vi "S4GUI_001.vi"() -> ()   [LabVIEW 2018] (continued)
                # "obsType"
                n1586 = call-dynamic "Read AcquisitionD.vi"("error in (no error)"=w3637, "S4ACS_GUI in"=w3638) -> ("error out"=w3627:errorcluster, "Acquisition.lvclass"=w3626:refnum<class "Acquisition.lvclass">, "S4ACS_GUI out"=w3616:refnum<class "S4GUI.lvclass">)  [unwired: 7 in]
                n1587 = local read "Exptime ch4"() -> (w3588:dbl)
                n1588 = call-dynamic "Read Channel.vi"("error in (no error)"=w3627, "Acquisition in"=w3626) -> ("error out"=w3624:errorcluster, "Channel.lvclass"=w3625:refnum<class "Channel.lvclass">, "Acquisition out"=w3615:refnum<class "Acquisition.lvclass">)  [unwired: 7 in]
                n1589 = call-dynamic "Read Interface.vi"("error in (no error)"=w3624, "Channel in"=w3625) -> ("error out"=w3633:errorcluster, "Interface.lvclass"=w3622:refnum<class "Interface.lvclass">, "Channel out"=w3623:refnum<class "Channel.lvclass">)  [unwired: 7 in]
                n1590 = call "Write Exposure Time.vi"("error in (no error)"=w3633, "Exposure Time"=w3588, "Interface in"=w3622) -> ("error out"=w3590:errorcluster, "Interface out"=w3592:refnum<class "Interface.lvclass">)  [unwired: 7 in]
                n1591 = case shown="Default" w3587 {
                  tunnel: w3592 -> [w3640 w3645]
                  tunnel: [w3640 w3644] -> w3591
                  tunnel: [w3639 w3643] -> w3589
                  tunnel: w3590 -> [w3639 w3642]
                  tunnel: w3588 -> [_ w3641]
                  frame "ZERO" {
                  }
                  frame Default {
                    n1592 = call-dynamic "Write prev ExpTime.vi"("error in (no error)"=w3642, "prev ExpTime"=w3641, "Interface in"=w3645) -> ("error out"=w3643:errorcluster, "Interface out"=w3644:refnum<class "Interface.lvclass">)  [unwired: 7 in]
                  }
                }
                n1593 = call-dynamic "Write Suffix.vi"("error in (no error)"=w3589, "Suffix"=w3634, "Interface in"=w3591) -> ("error out"=w3632:errorcluster, "Interface out"=w3621:refnum<class "Interface.lvclass">)  [unwired: 7 in]
                n1594 = call-dynamic "Write ObsType.vi"("error in (no error)"=w3632, "ObsType"=w3607, "Interface in"=w3621) -> ("error out"=w3631:errorcluster, "Interface out"=w3620:refnum<class "Interface.lvclass">)  [unwired: 7 in]
                n1595 = call-dynamic "Write Object.vi"("error in (no error)"=w3631, "Object"=w3606, "Interface in"=w3620) -> ("error out"=w3630:errorcluster, "Interface out"=w3619:refnum<class "Interface.lvclass">)  [unwired: 7 in]
                n1596 = call-dynamic "Write Comments.vi"("error in (no error)"=w3630, "Comments"=w3608, "Interface in"=w3619) -> ("error out"=w3629:errorcluster, "Interface out"=w3618:refnum<class "Interface.lvclass">)  [unwired: 7 in]
                n1597 = call-dynamic "Write DS9.vi"("error in (no error)"=w3629, "DS9"="F", "Interface in"=w3618) -> ("error out"=w3603:errorcluster, "Interface out"=w3605:refnum<class "Interface.lvclass">)  [unwired: 7 in]
                n1598 = property on="Exposure Time ch4" class="Slide (strict)"("Scale.Maximum"=w3588, "Scale.Minimum"=0.0 ("Scale.Range:Minimum")) -> ()  [unwired: 2 in, 2 out]
                n1599 = local read "Exp ch4"() -> (w3611:u32)
                n1600 = call-dynamic "Write Observer.vi"("error in (no error)"=w3603, "Observer"=w3601, "Interface in"=w3605) -> ("error out"=w3602:errorcluster, "Interface out"=w3604:refnum<class "Interface.lvclass">)  [unwired: 7 in]
                n1601 = property on="Exposure Done ch4" class="Slide (strict)"("Scale.Maximum"=w3611, "Scale.Minimum"=0.0 ("Scale.Range:Minimum")) -> ()  [unwired: 2 in, 2 out]
                n1602 = call-dynamic "Write # Images.vi"("error in (no error)"=w3602, "# Images"=w3611, "Interface in"=w3604) -> ("error out"=w3628:errorcluster, "Interface out"=w3617:refnum<class "Interface.lvclass">)  [unwired: 7 in]
                n1603 = call-dynamic "Write Interface.vi"("error in (no error)"=w3628, "Interface.lvclass"=w3617, "Channel in"=w3623) -> ("error out"=w3600:errorcluster, "Channel out"=w3599:refnum<class "Channel.lvclass">)  [unwired: 7 in]
                n1604 = call-dynamic "Write ciclos.vi"("error in (no error)"=w3600, "ciclos"=w3598, "Channel in"=w3599) -> ("error out"=w3596:errorcluster, "Channel out"=w3597:refnum<class "Channel.lvclass">)  [unwired: 7 in]
                n1605 = call-dynamic "Write sequencias.vi"("error in (no error)"=w3596, "sequencias"=w3593, "Channel in"=w3597) -> ("error out"=w3595:errorcluster, "Channel out"=w3594:refnum<class "Channel.lvclass">)  [unwired: 7 in]
                n1606 = call-dynamic "Write Channel.vi"("error in (no error)"=w3595, "Channel.lvclass"=w3594, "Acquisition in"=w3615) -> ("error out"=w3613:errorcluster, "Acquisition out"=w3614:refnum<class "Acquisition.lvclass">)  [unwired: 7 in]
                n1607 = call-dynamic "Write AcquisitionD.vi"("error in (no error)"=w3613, "Acquisition.lvclass"=w3614, "S4ACS_GUI in"=w3616) -> ("error out"=w3635:errorcluster, "S4ACS_GUI out"=w3636:refnum<class "S4GUI.lvclass">)  [unwired: 7 in]
              }
            }
            n1608 = call-dynamic "Write sequencias.vi"("error in (no error)"=w3387, "sequencias"=w3383, "S4GUI in"=w3385) -> ("error out"=w3386:errorcluster, "S4GUI out"=w3384:refnum<class "S4GUI.lvclass">)  [unwired: 7 in]
            n1609 = call-dynamic "Write ciclos.vi"("error in (no error)"=w3386, "ciclos"=w3388, "S4ACS_GUI in"=w3384) -> ("error out"=w3390:errorcluster, "S4ACS_GUI out"=w3392:refnum<class "S4GUI.lvclass">)  [unwired: 7 in]
            n1610 = property on="#Cycles Done" class="Slide (strict)"("Scale.Maximum"=w3388, "Scale.Minimum"=0.0 ("Scale.Range:Minor Increment")) -> ()  [unwired: 2 in, 2 out]
            n1611 = call-dynamic "Write TotalCiclos.vi"("error in (no error)"=w3390, "TotalCiclos"=w3388, "S4GUI in"=w3392) -> ("error out"=w3389:errorcluster, "S4GUI out"=w3391:refnum<class "S4GUI.lvclass">)  [unwired: 7 in]
          }
        }
        n1612 = property on="Pause SM" class="Bool"(error in=w3251, "DisabledEnum"=T7."Enabled" ("Disabled")) -> (error out=w3250:errorcluster)  [unwired: 1 in, 1 out]
      }
      event "# Cycles": Value Change {
        w3646 = 0.0 ("Scale.Range:Minor Increment")
        n1613 = event-data() -> ("NewVal"=w3647:u32)  [unwired: 1 in]
        n1614 = call-dynamic "Write ciclos.vi"("error in (no error)"=w3650, "ciclos"=w3647, "S4ACS_GUI in"=w3651) -> ("error out"=w3649:errorcluster, "S4ACS_GUI out"=w3648:refnum<class "S4GUI.lvclass">)  [unwired: 7 in]
        n1615 = property on="#Cycles Done" class="Slide (strict)"("Scale.Maximum"=w3647, "Scale.Minimum"=w3646) -> ()  [unwired: 2 in, 2 out]
        n1616 = property on="Cycles Done ch2" class="Slide (strict)"("Scale.Maximum"=w3647, "Scale.Minimum"=w3646) -> ()  [unwired: 2 in, 2 out]
        n1617 = property on="Cycles Done ch4" class="Slide (strict)"("Scale.Maximum"=w3647, "Scale.Minimum"=w3646) -> ()  [unwired: 2 in, 2 out]
        n1618 = property on="Cycles Done ch1" class="Slide (strict)"("Scale.Maximum"=w3647, "Scale.Minimum"=w3646) -> ()  [unwired: 2 in, 2 out]
        n1619 = property on="Cycles Done ch3" class="Slide (strict)"("Scale.Maximum"=w3647, "Scale.Minimum"=w3646) -> ()  [unwired: 2 in, 2 out]
      }
      event "AllConfig": Value Change {
        n1620 = event-data() -> ()  [unwired: 1 in, 6 out]
        n1621 = call "Read Instrument.lvclass.vi"("error in (no error)"=w3656, "S4ACS_GUI in"=w3657) -> ("error out"=w3736:errorcluster, "Instrument.lvclass"=w3703:refnum<class "Instrument.lvclass">, "S4ACS_GUI out"=w3734:refnum<class "S4GUI.lvclass">)  [unwired: 7 in]
        n1622 = call "Read ASEL.vi"("error in (no error)"=w3736, "Instrument in"=w3703) -> ("error out"=w3728:errorcluster, "Opt_Selector.lvclass"=w3727:refnum<class "Opt_Selector.lvclass">, "Instrument out"=w3735:refnum<class "Instrument.lvclass">)  [unwired: 7 in]
        n1623 = call-dynamic "Read State Machine.vi"("error in (no error)"=w3728, "Device in"=w3727) -> ("error out"=w3731:errorcluster, "State Machine.lvclass"=w3733:refnum<class "State Machine.lvclass">, "Device out"=w3725:refnum<class "Opt_Selector.lvclass">)  [unwired: 7 in]
        n1624 = call "Next State.vi"("error in (no error)"=w3731, "New_State"=1, "State Machine in"=w3733) -> ("error out"=w3730:errorcluster, "State Machine out"=w3729:refnum<class "State Machine.lvclass">)  [unwired: 7 in]
        n1625 = call-dynamic "Write State Machine.vi"("error in (no error)"=w3730, "State Machine.lvclass"=w3729, "Device in"=w3725) -> ("error out"=w3724:errorcluster, "Device out"=w3726:refnum<class "Opt_Selector.lvclass">)  [unwired: 7 in]
        n1626 = call "Write ASEL.vi"("error in (no error)"=w3724, "Opt_Selector.lvclass"=w3726, "Instrument in"=w3735) -> ("error out"=w3686:errorcluster, "Instrument out"=w3702:refnum<class "Instrument.lvclass">)  [unwired: 7 in]
        n1627 = call "Read CALW.vi"("error in (no error)"=w3686, "Instrument in"=w3702) -> ("error out"=w3719:errorcluster, "Opt_Selector.lvclass"=w3720:refnum<class "Opt_Selector.lvclass">, "Instrument out"=w3701:refnum<class "Instrument.lvclass">)  [unwired: 7 in]
        n1628 = call-dynamic "Read State Machine.vi"("error in (no error)"=w3719, "Device in"=w3720) -> ("error out"=w3716:errorcluster, "State Machine.lvclass"=w3714:refnum<class "State Machine.lvclass">, "Device out"=w3722:refnum<class "Opt_Selector.lvclass">)  [unwired: 7 in]
        n1629 = call "Next State.vi"("error in (no error)"=w3716, "New_State"=1, "State Machine in"=w3714) -> ("error out"=w3717:errorcluster, "State Machine out"=w3718:refnum<class "State Machine.lvclass">)  [unwired: 7 in]
        n1630 = call-dynamic "Write State Machine.vi"("error in (no error)"=w3717, "State Machine.lvclass"=w3718, "Device in"=w3722) -> ("error out"=w3723:errorcluster, "Device out"=w3721:refnum<class "Opt_Selector.lvclass">)  [unwired: 7 in]
        n1631 = call "Write CALW.vi"("error in (no error)"=w3723, "Opt_Selector.lvclass"=w3721, "Instrument in"=w3701) -> ("error out"=w3685:errorcluster, "Instrument out"=w3700:refnum<class "Instrument.lvclass">)  [unwired: 7 in]
        n1632 = call "Read WPSEL.vi"("error in (no error)"=w3685, "Instrument in"=w3700) -> ("error out"=w3708:errorcluster, "Opt_Selector.lvclass"=w3707:refnum<class "Opt_Selector.lvclass">, "Instrument out"=w3699:refnum<class "Instrument.lvclass">)  [unwired: 7 in]
        n1633 = call-dynamic "Read State Machine.vi"("error in (no error)"=w3708, "Device in"=w3707) -> ("error out"=w3711:errorcluster, "State Machine.lvclass"=w3713:refnum<class "State Machine.lvclass">, "Device out"=w3705:refnum<class "Opt_Selector.lvclass">)  [unwired: 7 in]
        n1634 = call "Next State.vi"("error in (no error)"=w3711, "New_State"=1, "State Machine in"=w3713) -> ("error out"=w3710:errorcluster, "State Machine out"=w3709:refnum<class "State Machine.lvclass">)  [unwired: 7 in]
        n1635 = call-dynamic "Write State Machine.vi"("error in (no error)"=w3710, "State Machine.lvclass"=w3709, "Device in"=w3705) -> ("error out"=w3704:errorcluster, "Device out"=w3706:refnum<class "Opt_Selector.lvclass">)  [unwired: 7 in]
        n1636 = call "Write WPSEL.vi"("error in (no error)"=w3704, "Opt_Selector.lvclass"=w3706, "Instrument in"=w3699) -> ("error out"=w3684:errorcluster, "Instrument out"=w3688:refnum<class "Instrument.lvclass">)  [unwired: 7 in]
        n1637 = call "Read WPROT.vi"("error in (no error)"=w3684, "Instrument in"=w3688) -> ("error out"=w3694:errorcluster, "Opt_Selector.lvclass"=w3695:refnum<class "Opt_Selector.lvclass">, "Instrument out"=w3687:refnum<class "Instrument.lvclass">)  [unwired: 7 in]
        n1638 = call-dynamic "Read State Machine.vi"("error in (no error)"=w3694, "Device in"=w3695) -> ("error out"=w3691:errorcluster, "State Machine.lvclass"=w3689:refnum<class "State Machine.lvclass">, "Device out"=w3697:refnum<class "Opt_Selector.lvclass">)  [unwired: 7 in]
        n1639 = call "Next State.vi"("error in (no error)"=w3691, "New_State"=1, "State Machine in"=w3689) -> ("error out"=w3692:errorcluster, "State Machine out"=w3693:refnum<class "State Machine.lvclass">)  [unwired: 7 in]
        n1640 = call-dynamic "Write State Machine.vi"("error in (no error)"=w3692, "State Machine.lvclass"=w3693, "Device in"=w3697) -> ("error out"=w3698:errorcluster, "Device out"=w3696:refnum<class "Opt_Selector.lvclass">)  [unwired: 7 in]
        n1641 = call "Write WPROT.vi"("error in (no error)"=w3698, "Opt_Selector.lvclass"=w3696, "Instrument in"=w3687) -> ("error out"=w3660:errorcluster, "Instrument out"=w3661:refnum<class "Instrument.lvclass">)  [unwired: 7 in]
        n1642 = call "Read GMIR.vi"("error in (no error)"=w3660, "Instrument in"=w3661) -> ("error out"=w3679:errorcluster, "Opt_Continuous.lvclass"=w3680:refnum<class "Opt_Continuous.lvclass">, "Instrument out"=w3673:refnum<class "Instrument.lvclass">)  [unwired: 7 in]
        n1643 = call-dynamic "Read State Machine.vi"("error in (no error)"=w3679, "Device in"=w3680) -> ("error out"=w3676:errorcluster, "State Machine.lvclass"=w3674:refnum<class "State Machine.lvclass">, "Device out"=w3682:refnum<class "Opt_Continuous.lvclass">)  [unwired: 7 in]
        n1644 = call "Next State.vi"("error in (no error)"=w3676, "New_State"=1, "State Machine in"=w3674) -> ("error out"=w3677:errorcluster, "State Machine out"=w3678:refnum<class "State Machine.lvclass">)  [unwired: 7 in]
        n1645 = call-dynamic "Write State Machine.vi"("error in (no error)"=w3677, "State Machine.lvclass"=w3678, "Device in"=w3682) -> ("error out"=w3683:errorcluster, "Device out"=w3681:refnum<class "Opt_Continuous.lvclass">)  [unwired: 7 in]
        n1646 = call "Write GMIR.vi"("error in (no error)"=w3683, "Opt_Continuous.lvclass"=w3681, "Instrument in"=w3673) -> ("error out"=w3658:errorcluster, "Instrument out"=w3659:refnum<class "Instrument.lvclass">)  [unwired: 7 in]
        n1647 = call "Read GFOC.vi"("error in (no error)"=w3658, "Instrument in"=w3659) -> ("error out"=w3668:errorcluster, "Opt_Continuous.lvclass"=w3669:refnum<class "Opt_Continuous.lvclass">, "Instrument out"=w3662:refnum<class "Instrument.lvclass">)  [unwired: 7 in]
        n1648 = call-dynamic "Read State Machine.vi"("error in (no error)"=w3668, "Device in"=w3669) -> ("error out"=w3665:errorcluster, "State Machine.lvclass"=w3663:refnum<class "State Machine.lvclass">, "Device out"=w3671:refnum<class "Opt_Continuous.lvclass">)  [unwired: 7 in]
        n1649 = call "Next State.vi"("error in (no error)"=w3665, "New_State"=1, "State Machine in"=w3663) -> ("error out"=w3666:errorcluster, "State Machine out"=w3667:refnum<class "State Machine.lvclass">)  [unwired: 7 in]
        n1650 = call-dynamic "Write State Machine.vi"("error in (no error)"=w3666, "State Machine.lvclass"=w3667, "Device in"=w3671) -> ("error out"=w3672:errorcluster, "Device out"=w3670:refnum<class "Opt_Continuous.lvclass">)  [unwired: 7 in]
        n1651 = call "Write GFOC.vi"("error in (no error)"=w3672, "Opt_Continuous.lvclass"=w3670, "Instrument in"=w3662) -> ("error out"=w3654:errorcluster, "Instrument out"=w3655:refnum<class "Instrument.lvclass">)  [unwired: 7 in]
        n1652 = call "Write Instrument.lvclass.vi"("error in (no error)"=w3654, "Instrument.lvclass"=w3655, "S4ACS_GUI in"=w3734) -> ("error out"=w3653:errorcluster, "S4ACS_GUI out"=w3652:refnum<class "S4GUI.lvclass">)  [unwired: 7 in]
      }
      event "Tab Acq Type": Value Change {
        # "Tab for choosing EXPOSURE MODE: Object, Dflat, Sflat, Dark, Zero, Focus"
        n1653 = event-data() -> ("NewVal"=w3743:T1)  [unwired: 1 in]
        n1654 = local read "Observer"() -> (w3739:string)
        n1655 = case shown="\"ZERO\"" w3743 {
          tunnel: ["OBJECT" "FLAT" "FLAT" "DARK" "ZERO" "FOCUS"] -> w3737
          tunnel: [w3779 w3783 w3787 w3791 w3795 w3799] -> w3742
          tunnel: [w3778 w3782 w3786 w3790 w3794 w3798] -> w3741
          tunnel: [w3777 w3781 w3785 w3789 w3793 w3797] -> w3740
          frame "OBJECT", Default {
            n1656 = local read "Object_obj"() -> (w3779:string)
            n1657 = local read "OBJECT Comments"() -> (w3777:string)
            n1658 = local read "object suffix"() -> (w3778:string)
          }
          frame "DFLAT" {
            n1659 = local read "DFLAT Comments"() -> (w3781:string)
            n1660 = local read "Object_dflat"() -> (w3783:string)
            n1661 = local read "dflat suffix"() -> (w3782:string)
          }
          frame "SFLAT" {
            n1662 = local read "SFLAT Comments"() -> (w3785:string)
            n1663 = local read "Object_sflat"() -> (w3787:string)
            n1664 = local read "sflat suffix"() -> (w3786:string)
          }
          frame "DARK" {
            n1665 = local read "Object_dark"() -> (w3791:string)
            n1666 = local read "dark suffix"() -> (w3790:string)
            n1667 = local read "DARK Comments"() -> (w3789:string)
          }
          frame "ZERO" {
            n1668 = local read "ZERO Comments"() -> (w3793:string)
            n1669 = local read "Object_zero"() -> (w3795:string)
            n1670 = local read "zero suffix"() -> (w3794:string)
          }
          frame "FOCUS" {
            n1671 = local read "FOCUS Comments"() -> (w3797:string)
            n1672 = local read "Object_focus"() -> (w3799:string)
            n1673 = local read "focus suffix"() -> (w3798:string)
          }
        }
        n1674 = call-dynamic "Write ExpMode.vi"("error in (no error)"=w3746, "ExpMode"=w3743, "S4GUI in"=w3747) -> ("error out"=w3744:errorcluster, "S4GUI out"=w3745:refnum<class "S4GUI.lvclass">)  [unwired: 7 in]
        n1675 = call-dynamic "Read AcquisitionC.vi"("error in (no error)"=w3744, "S4ACS_GUI in"=w3745) -> ("error out"=w3750:errorcluster, "Acquisition.lvclass"=w3751:refnum<class "Acquisition.lvclass">)  [unwired: 7 in, 1 out]
        n1676 = call-dynamic "Read AcquisitionA.vi"("error in (no error)"=w3744, "S4ACS_GUI in"=w3745) -> ("error out"=w3754:errorcluster, "Acquisition.lvclass"=w3755:refnum<class "Acquisition.lvclass">, "S4ACS_GUI out"=w3776:refnum<class "S4GUI.lvclass">)  [unwired: 7 in]
        n1677 = call "Read AcquisitionB.vi"("error in (no error)"=w3744, "S4ACS_GUI in"=w3745) -> ("error out"=w3752:errorcluster, "Acquisition.lvclass"=w3753:refnum<class "Acquisition.lvclass">)  [unwired: 7 in, 1 out]
        n1678 = call-dynamic "Read AcquisitionD.vi"("error in (no error)"=w3744, "S4ACS_GUI in"=w3745) -> ("error out"=w3748:errorcluster, "Acquisition.lvclass"=w3749:refnum<class "Acquisition.lvclass">)  [unwired: 7 in, 1 out]
        n1679 = To Lower Case(string=w3741) -> (all lower case string=w3738:string)
        n1680 = case shown="\"ZERO\"" w3743 {
          tunnel: [w3834 w4159 w4512] -> w3775
          tunnel: [w3833 w4158 w4511] -> w3774
          tunnel: [w3832 w4157 w4510] -> w3770
          tunnel: [w3831 w4156 w4509] -> w3769
          tunnel: [w3830 w4155 w4508] -> w3759
          tunnel: [w3829 w4154 w4507] -> w3758
          tunnel: [w3828 w4153 w4506] -> w3757
          tunnel: [w3827 w4152 w4505] -> w3756
          tunnel: w3755 -> [w3826 w4151 w4504]
          tunnel: w3754 -> [w3825 w4150 w4503]
          tunnel: w3753 -> [w3811 w4137 w4490]
          tunnel: w3752 -> [w3810 w4136 w4489]
          tunnel: w3751 -> [w3809 w4135 w4488]
          tunnel: w3750 -> [w3808 w4134 w4487]
          tunnel: w3749 -> [w3807 w4133 w4486]
          tunnel: w3748 -> [w3806 w4132 w4485]
          tunnel: w3742 -> [w3803 w4131 w4484]
          tunnel: w3740 -> [w3804 w4130 w4483]
          tunnel: w3739 -> [w3805 w4129 w4482]
          tunnel: w3738 -> [w3802 w4128 w4481]
          tunnel: w3737 -> [w3801 w4127 w4480]
          frame "ZERO" {
            w3824 = 1e-05 ("Exptime ch1")
            # "ZERO: EXPTIME=1E-5 (mandatory), shutter automatically closed, save current FRAME_TRANSFER (prev_FT) and reset FRAME_TRANSFER."
            n1681 = call "Read connection.vi"("error in (no error)"=w3808, "Server in"=w3809) -> ("error out"=w3816:errorcluster, "connection"=w3815:bool, "Server out"=w3817:refnum<class "Acquisition.lvclass">)  [unwired: 7 in]
            n1682 = call "Read connection.vi"("error in (no error)"=w3810, "Server in"=w3811) -> ("error out"=w3819:errorcluster, "connection"=w3818:bool, "Server out"=w3820:refnum<class "Acquisition.lvclass">)  [unwired: 7 in]
            n1683 = call "Read connection.vi"("error in (no error)"=w3825, "Server in"=w3826) -> ("error out"=w3822:errorcluster, "connection"=w3821:bool, "Server out"=w3823:refnum<class "Acquisition.lvclass">)  [unwired: 7 in]
            n1684 = call "Read connection.vi"("error in (no error)"=w3806, "Server in"=w3807) -> ("error out"=w3813:errorcluster, "connection"=w3812:bool, "Server out"=w3814:refnum<class "Acquisition.lvclass">)  [unwired: 7 in]
            n1685 = case shown="True" w3818 {
              tunnel: w3820 -> [w3982 w4022]
              tunnel: w3819 -> [w3981 w4021]
              tunnel: [w3982 w4020] -> w3832
              tunnel: [w3981 w4019] -> w3831
              tunnel: w3805 -> [_ w3998]
              tunnel: w3804 -> [_ w3997]
              tunnel: w3803 -> [_ w3996]
              tunnel: w3802 -> [_ w3989]
              tunnel: w3801 -> [_ w3988]
              frame False {
              }
              frame True {
                # "nome do arquivo .cfg"
                # "seção no arquivo .cfg"
                n1686 = call-dynamic "Read Channel.vi"("error in (no error)"=w4021, "Acquisition in"=w4022) -> ("error out"=w4026:errorcluster, "Channel.lvclass"=w4025:refnum<class "Channel.lvclass">, "Acquisition out"=w4024:refnum<class "Acquisition.lvclass">)  [unwired: 7 in]
                n1687 = call-dynamic "Read Interface.vi"("error in (no error)"=w4026, "Channel in"=w4025) -> ("error out"=w3985:errorcluster, "Interface.lvclass"=w3986:refnum<class "Interface.lvclass">, "Channel out"=w4023:refnum<class "Channel.lvclass">)  [unwired: 7 in]
                n1688 = call-dynamic "Write restoreExpTime.vi"("error in (no error)"=w3985, "restoreExpTime"=TRUE, "Interface in"=w3986) -> ("error out"=w3983:errorcluster, "Interface out"=w3984:refnum<class "Interface.lvclass">)  [unwired: 7 in]
                n1689 = call-dynamic "Get CCD_Config.vi"("error in (no error)"=w3983, "Interface in"=w3984) -> ("error out"=w3992:errorcluster, "output cluster"=w3995:T24, "Interface out"=w3993:refnum<class "Interface.lvclass">)  [unwired: 7 in]
                n1690 = stacked-sequence {
                  tunnel: [_ w4052] -> w4030
                  tunnel: w3995 -> [_ w4051]
                  tunnel: w3995 -> [w4049 _]
                  tunnel: [w4048 _] -> w3990
                  frame #0 {
                    n1691 = Unbundle By Name(w4049) -> ("FRAME_TRANSFER"=w4048:bool)
                  }
                  frame #1 {
                    # "closed"
                    n1692 = Bundle By Name(cluster=w4051, "SHUTTER_MODE"=u8 2, "FRAME_TRANSFER"=FALSE) -> (w4052:T24)
                  }
                }
                n1693 = call-dynamic "Write PREV_FT.vi"("error in (no error)"=w3992, "PREV_FT"=w3990, "Interface in"=w3993) -> ("error out"=w3991:errorcluster, "Interface out"=w3994:refnum<class "Interface.lvclass">)  [unwired: 7 in]
                n1694 = call-dynamic "Set CCD_Config.vi"("error in (no error)"=w3991, "input cluster"=w4030, "Interface in"=w3994) -> ("error out"=w4029:errorcluster, "Interface out"=w4031:refnum<class "Interface.lvclass">)  [unwired: 7 in]
                n1695 = Flatten To String(anything=w4030, error in (no error)=w4029) -> (data string=w4027:string, error out=w4028:errorcluster)  [unwired: 2 in, 1 out]
                n1696 = call "Write flatted cluster.vi"("error in (no error)"=w4028, "flatted cluster"=w4027, "Interface in"=w4031) -> ("error out"=w4033:errorcluster, "Interface out"=w4032:refnum<class "Interface.lvclass">)  [unwired: 7 in]
                n1697 = call-dynamic "Write Interface.vi"("error in (no error)"=w4033, "Interface.lvclass"=w4032, "Channel in"=w4023) -> ("error out"=w4038:errorcluster, "Channel out"=w4039:refnum<class "Channel.lvclass">)  [unwired: 7 in]
                n1698 = call "Write section_name.vi"("error in (no error)"=w4038, "section_name"="CCD_ACS2", "Channel in"=w4039) -> ("error out"=w4037:errorcluster, "Channel out"=w4042:refnum<class "Channel.lvclass">)  [unwired: 7 in]
                n1699 = call-dynamic "save config.vi"("error in (no error)"=w4037, "file config"="lastsaved.cfg", "Channel in"=w4042) -> ("error out"=w4001:errorcluster, "Channel out"=w4002:refnum<class "Channel.lvclass">)  [unwired: 7 in]
                n1700 = local read "Filter2"() -> (w4003:u8)
                n1701 = call-dynamic "Write Filter.vi"("error in (no error)"=w4001, "Filter"=w4003, "Channel in"=w4002) -> ("error out"=w4010:errorcluster, "Channel out"=w4011:refnum<class "Channel.lvclass">)  [unwired: 7 in]
                n1702 = call-dynamic "Read Interface.vi"("error in (no error)"=w4010, "Channel in"=w4011) -> ("error out"=w4008:errorcluster, "Interface.lvclass"=w4013:refnum<class "Interface.lvclass">, "Channel out"=w4012:refnum<class "Channel.lvclass">)  [unwired: 7 in]
                n1703 = call-dynamic "Write Suffix.vi"("error in (no error)"=w4008, "Suffix"=w3989, "Interface in"=w4013) -> ("error out"=w4004:errorcluster, "Interface out"=w4014:refnum<class "Interface.lvclass">)  [unwired: 7 in]
                n1704 = call-dynamic "Write ObsType.vi"("error in (no error)"=w4004, "ObsType"=w3988, "Interface in"=w4014) -> ("error out"=w4005:errorcluster, "Interface out"=w4015:refnum<class "Interface.lvclass">)  [unwired: 7 in]
                n1705 = call-dynamic "Write Object.vi"("error in (no error)"=w4005, "Object"=w3996, "Interface in"=w4015) -> ("error out"=w4006:errorcluster, "Interface out"=w4016:refnum<class "Interface.lvclass">)  [unwired: 7 in]
                n1706 = call-dynamic "Write Comments.vi"("error in (no error)"=w4006, "Comments"=w3997, "Interface in"=w4016) -> ("error out"=w4007:errorcluster, "Interface out"=w4017:refnum<class "Interface.lvclass">)  [unwired: 7 in]
                n1707 = call-dynamic "Write Observer.vi"("error in (no error)"=w4007, "Observer"=w3998, "Interface in"=w4017) -> ("error out"=w4009:errorcluster, "Interface out"=w4018:refnum<class "Interface.lvclass">)  [unwired: 7 in]
                n1708 = call-dynamic "Write Interface.vi"("error in (no error)"=w4009, "Interface.lvclass"=w4018, "Channel in"=w4012) -> ("error out"=w4000:errorcluster, "Channel out"=w3999:refnum<class "Channel.lvclass">)  [unwired: 7 in]
                n1709 = call-dynamic "Read State Machine.vi"("error in (no error)"=w4000, "Device in"=w3999) -> ("error out"=w4034:errorcluster, "State Machine.lvclass"=w4044:refnum<class "State Machine.lvclass">, "Device out"=w4043:refnum<class "Channel.lvclass">)  [unwired: 7 in]
                n1710 = call-dynamic "Write State.vi"("error in (no error)"=w4034, "State"=60, "State Machine in"=w4044) -> ("error out"=w4035:errorcluster, "State Machine out"=w4045:refnum<class "State Machine.lvclass">)  [unwired: 7 in]
                n1711 = call-dynamic "Write State Machine.vi"("error in (no error)"=w4035, "State Machine.lvclass"=w4045, "Device in"=w4043) -> ("error out"=w4047:errorcluster, "Device out"=w4046:refnum<class "Channel.lvclass">)  [unwired: 7 in]
                n1712 = call-dynamic "Write Channel.vi"("error in (no error)"=w4047, "Channel.lvclass"=w4046, "Acquisition in"=w4024) -> ("error out"=w4019:errorcluster, "Acquisition out"=w4020:refnum<class "Acquisition.lvclass">)  [unwired: 7 in]
              }
            }
            n1713 = case shown="True" w3821 {
              tunnel: [w4054 w4116] -> w3833
              tunnel: [w4055 w4115] -> w3834
              tunnel: w3823 -> [w4055 w4093]
              tunnel: w3822 -> [w4054 w4092]
              tunnel: w3805 -> [_ w4071]
              tunnel: w3804 -> [_ w4070]
              tunnel: w3803 -> [_ w4069]
              tunnel: w3802 -> [_ w4062]
              tunnel: w3801 -> [_ w4061]
              frame False {
              }
              frame True {
                # "nome do arquivo .cfg"
                # "seção no arquivo .cfg"
                n1714 = call-dynamic "Read Channel.vi"("error in (no error)"=w4092, "Acquisition in"=w4093) -> ("error out"=w4117:errorcluster, "Channel.lvclass"=w4118:refnum<class "Channel.lvclass">, "Acquisition out"=w4119:refnum<class "Acquisition.lvclass">)  [unwired: 7 in]
                n1715 = call-dynamic "Read Interface.vi"("error in (no error)"=w4117, "Channel in"=w4118) -> ("error out"=w4058:errorcluster, "Interface.lvclass"=w4060:refnum<class "Interface.lvclass">, "Channel out"=w4120:refnum<class "Channel.lvclass">)  [unwired: 7 in]
                n1716 = call-dynamic "Write restoreExpTime.vi"("error in (no error)"=w4058, "restoreExpTime"=TRUE, "Interface in"=w4060) -> ("error out"=w4057:errorcluster, "Interface out"=w4059:refnum<class "Interface.lvclass">)  [unwired: 7 in]
                n1717 = call-dynamic "Get CCD_Config.vi"("error in (no error)"=w4057, "Interface in"=w4059) -> ("error out"=w4066:errorcluster, "output cluster"=w4064:T24, "Interface out"=w4068:refnum<class "Interface.lvclass">)  [unwired: 7 in]
                n1718 = stacked-sequence {
                  tunnel: [_ w4126] -> w4111
                  tunnel: w4064 -> [_ w4123]
                  tunnel: w4064 -> [w4122 _]
                  tunnel: [w4121 _] -> w4063
                  frame #0 {
                    n1719 = Unbundle By Name(w4122) -> ("FRAME_TRANSFER"=w4121:bool)
                  }
                  frame #1 {
                    # "closed"
                    n1720 = Bundle By Name(cluster=w4123, "SHUTTER_MODE"=u8 2, "FRAME_TRANSFER"=FALSE) -> (w4126:T24)
                  }
                }
                n1721 = call-dynamic "Write PREV_FT.vi"("error in (no error)"=w4066, "PREV_FT"=w4063, "Interface in"=w4068) -> ("error out"=w4065:errorcluster, "Interface out"=w4067:refnum<class "Interface.lvclass">)  [unwired: 7 in]
                n1722 = call-dynamic "Set CCD_Config.vi"("error in (no error)"=w4065, "input cluster"=w4111, "Interface in"=w4067) -> ("error out"=w4112:errorcluster, "Interface out"=w4110:refnum<class "Interface.lvclass">)  [unwired: 7 in]
                n1723 = Flatten To String(anything=w4111, error in (no error)=w4112) -> (data string=w4114:string, error out=w4113:errorcluster)  [unwired: 2 in, 1 out]
                n1724 = call "Write flatted cluster.vi"("error in (no error)"=w4113, "flatted cluster"=w4114, "Interface in"=w4110) -> ("error out"=w4108:errorcluster, "Interface out"=w4109:refnum<class "Interface.lvclass">)  [unwired: 7 in]
                n1725 = call-dynamic "Write Interface.vi"("error in (no error)"=w4108, "Interface.lvclass"=w4109, "Channel in"=w4120) -> ("error out"=w4103:errorcluster, "Channel out"=w4102:refnum<class "Channel.lvclass">)  [unwired: 7 in]
                n1726 = call "Write section_name.vi"("error in (no error)"=w4103, "section_name"="CCD_ACS1", "Channel in"=w4102) -> ("error out"=w4104:errorcluster, "Channel out"=w4099:refnum<class "Channel.lvclass">)  [unwired: 7 in]
                n1727 = call-dynamic "save config.vi"("error in (no error)"=w4104, "file config"="lastsaved.cfg", "Channel in"=w4099) -> ("error out"=w4082:errorcluster, "Channel out"=w4083:refnum<class "Channel.lvclass">)  [unwired: 7 in]
                n1728 = local read "Filter1"() -> (w4084:u8)
                n1729 = call-dynamic "Write Filter.vi"("error in (no error)"=w4082, "Filter"=w4084, "Channel in"=w4083) -> ("error out"=w4091:errorcluster, "Channel out"=w4081:refnum<class "Channel.lvclass">)  [unwired: 7 in]
                n1730 = call-dynamic "Read Interface.vi"("error in (no error)"=w4091, "Channel in"=w4081) -> ("error out"=w4089:errorcluster, "Interface.lvclass"=w4080:refnum<class "Interface.lvclass">, "Channel out"=w4074:refnum<class "Channel.lvclass">)  [unwired: 7 in]
                n1731 = call-dynamic "Write Suffix.vi"("error in (no error)"=w4089, "Suffix"=w4062, "Interface in"=w4080) -> ("error out"=w4085:errorcluster, "Interface out"=w4079:refnum<class "Interface.lvclass">)  [unwired: 7 in]
                n1732 = call-dynamic "Write ObsType.vi"("error in (no error)"=w4085, "ObsType"=w4061, "Interface in"=w4079) -> ("error out"=w4086:errorcluster, "Interface out"=w4078:refnum<class "Interface.lvclass">)  [unwired: 7 in]
                n1733 = call-dynamic "Write Object.vi"("error in (no error)"=w4086, "Object"=w4069, "Interface in"=w4078) -> ("error out"=w4087:errorcluster, "Interface out"=w4077:refnum<class "Interface.lvclass">)  [unwired: 7 in]
                n1734 = call-dynamic "Write Comments.vi"("error in (no error)"=w4087, "Comments"=w4070, "Interface in"=w4077) -> ("error out"=w4088:errorcluster, "Interface out"=w4076:refnum<class "Interface.lvclass">)  [unwired: 7 in]
                n1735 = call-dynamic "Write Observer.vi"("error in (no error)"=w4088, "Observer"=w4071, "Interface in"=w4076) -> ("error out"=w4090:errorcluster, "Interface out"=w4075:refnum<class "Interface.lvclass">)  [unwired: 7 in]
                n1736 = call-dynamic "Write Interface.vi"("error in (no error)"=w4090, "Interface.lvclass"=w4075, "Channel in"=w4074) -> ("error out"=w4072:errorcluster, "Channel out"=w4073:refnum<class "Channel.lvclass">)  [unwired: 7 in]
                n1737 = call-dynamic "Read State Machine.vi"("error in (no error)"=w4072, "Device in"=w4073) -> ("error out"=w4107:errorcluster, "State Machine.lvclass"=w4097:refnum<class "State Machine.lvclass">, "Device out"=w4098:refnum<class "Channel.lvclass">)  [unwired: 7 in]
                n1738 = call-dynamic "Write State.vi"("error in (no error)"=w4107, "State"=60, "State Machine in"=w4097) -> ("error out"=w4106:errorcluster, "State Machine out"=w4096:refnum<class "State Machine.lvclass">)  [unwired: 7 in]
                n1739 = call-dynamic "Write State Machine.vi"("error in (no error)"=w4106, "State Machine.lvclass"=w4096, "Device in"=w4098) -> ("error out"=w4094:errorcluster, "Device out"=w4095:refnum<class "Channel.lvclass">)  [unwired: 7 in]
                n1740 = call-dynamic "Write Channel.vi"("error in (no error)"=w4094, "Channel.lvclass"=w4095, "Acquisition in"=w4119) -> ("error out"=w4116:errorcluster, "Acquisition out"=w4115:refnum<class "Acquisition.lvclass">)  [unwired: 7 in]
              }
            }
            n1741 = case shown="True" w3815 {
              tunnel: w3817 -> [w3909 w3949]
              tunnel: w3816 -> [w3908 w3948]
              tunnel: [w3909 w3947] -> w3830
              tunnel: [w3908 w3946] -> w3829
              tunnel: w3805 -> [_ w3925]
              tunnel: w3804 -> [_ w3924]
              tunnel: w3803 -> [_ w3923]
              tunnel: w3802 -> [_ w3916]
              tunnel: w3801 -> [_ w3915]
              frame False {
              }
              frame True {
                # "nome do arquivo .cfg"
                # "seção no arquivo .cfg"
                n1742 = call-dynamic "Read Channel.vi"("error in (no error)"=w3948, "Acquisition in"=w3949) -> ("error out"=w3953:errorcluster, "Channel.lvclass"=w3952:refnum<class "Channel.lvclass">, "Acquisition out"=w3951:refnum<class "Acquisition.lvclass">)  [unwired: 7 in]
                n1743 = call-dynamic "Read Interface.vi"("error in (no error)"=w3953, "Channel in"=w3952) -> ("error out"=w3911:errorcluster, "Interface.lvclass"=w3913:refnum<class "Interface.lvclass">, "Channel out"=w3950:refnum<class "Channel.lvclass">)  [unwired: 7 in]
                n1744 = call-dynamic "Write restoreExpTime.vi"("error in (no error)"=w3911, "restoreExpTime"=TRUE, "Interface in"=w3913) -> ("error out"=w3910:errorcluster, "Interface out"=w3912:refnum<class "Interface.lvclass">)  [unwired: 7 in]
                n1745 = call-dynamic "Get CCD_Config.vi"("error in (no error)"=w3910, "Interface in"=w3912) -> ("error out"=w3918:errorcluster, "output cluster"=w3922:T24, "Interface out"=w3921:refnum<class "Interface.lvclass">)  [unwired: 7 in]
                n1746 = stacked-sequence {
                  tunnel: [_ w3979] -> w3957
                  tunnel: w3922 -> [_ w3978]
                  tunnel: w3922 -> [w3976 _]
                  tunnel: [w3975 _] -> w3917
                  frame #0 {
                    n1747 = Unbundle By Name(w3976) -> ("FRAME_TRANSFER"=w3975:bool)
                  }
                  frame #1 {
                    # "closed"
                    n1748 = Bundle By Name(cluster=w3978, "SHUTTER_MODE"=u8 2, "FRAME_TRANSFER"=FALSE) -> (w3979:T24)
                  }
                }
                n1749 = call-dynamic "Write PREV_FT.vi"("error in (no error)"=w3918, "PREV_FT"=w3917, "Interface in"=w3921) -> ("error out"=w3919:errorcluster, "Interface out"=w3920:refnum<class "Interface.lvclass">)  [unwired: 7 in]
                n1750 = call-dynamic "Set CCD_Config.vi"("error in (no error)"=w3919, "input cluster"=w3957, "Interface in"=w3920) -> ("error out"=w3956:errorcluster, "Interface out"=w3958:refnum<class "Interface.lvclass">)  [unwired: 7 in]
                n1751 = Flatten To String(anything=w3957, error in (no error)=w3956) -> (data string=w3954:string, error out=w3955:errorcluster)  [unwired: 2 in, 1 out]
                n1752 = call "Write flatted cluster.vi"("error in (no error)"=w3955, "flatted cluster"=w3954, "Interface in"=w3958) -> ("error out"=w3960:errorcluster, "Interface out"=w3959:refnum<class "Interface.lvclass">)  [unwired: 7 in]
                n1753 = call-dynamic "Write Interface.vi"("error in (no error)"=w3960, "Interface.lvclass"=w3959, "Channel in"=w3950) -> ("error out"=w3965:errorcluster, "Channel out"=w3966:refnum<class "Channel.lvclass">)  [unwired: 7 in]
                n1754 = call "Write section_name.vi"("error in (no error)"=w3965, "section_name"="CCD_ACS3", "Channel in"=w3966) -> ("error out"=w3964:errorcluster, "Channel out"=w3969:refnum<class "Channel.lvclass">)  [unwired: 7 in]
                n1755 = call-dynamic "save config.vi"("error in (no error)"=w3964, "file config"="lastsaved.cfg", "Channel in"=w3969) -> ("error out"=w3927:errorcluster, "Channel out"=w3929:refnum<class "Channel.lvclass">)  [unwired: 7 in]
                n1756 = local read "Filter3"() -> (w3945:u8)
                n1757 = call-dynamic "Write Filter.vi"("error in (no error)"=w3927, "Filter"=w3945, "Channel in"=w3929) -> ("error out"=w3938:errorcluster, "Channel out"=w3937:refnum<class "Channel.lvclass">)  [unwired: 7 in]
                n1758 = call-dynamic "Read Interface.vi"("error in (no error)"=w3938, "Channel in"=w3937) -> ("error out"=w3940:errorcluster, "Interface.lvclass"=w3935:refnum<class "Interface.lvclass">, "Channel out"=w3936:refnum<class "Channel.lvclass">)  [unwired: 7 in]
                n1759 = call-dynamic "Write Suffix.vi"("error in (no error)"=w3940, "Suffix"=w3916, "Interface in"=w3935) -> ("error out"=w3944:errorcluster, "Interface out"=w3934:refnum<class "Interface.lvclass">)  [unwired: 7 in]
                n1760 = call-dynamic "Write ObsType.vi"("error in (no error)"=w3944, "ObsType"=w3915, "Interface in"=w3934) -> ("error out"=w3943:errorcluster, "Interface out"=w3933:refnum<class "Interface.lvclass">)  [unwired: 7 in]
                n1761 = call-dynamic "Write Object.vi"("error in (no error)"=w3943, "Object"=w3923, "Interface in"=w3933) -> ("error out"=w3942:errorcluster, "Interface out"=w3932:refnum<class "Interface.lvclass">)  [unwired: 7 in]
                n1762 = call-dynamic "Write Comments.vi"("error in (no error)"=w3942, "Comments"=w3924, "Interface in"=w3932) -> ("error out"=w3941:errorcluster, "Interface out"=w3931:refnum<class "Interface.lvclass">)  [unwired: 7 in]
                n1763 = call-dynamic "Write Observer.vi"("error in (no error)"=w3941, "Observer"=w3925, "Interface in"=w3931) -> ("error out"=w3939:errorcluster, "Interface out"=w3930:refnum<class "Interface.lvclass">)  [unwired: 7 in]
                n1764 = call-dynamic "Write Interface.vi"("error in (no error)"=w3939, "Interface.lvclass"=w3930, "Channel in"=w3936) -> ("error out"=w3926:errorcluster, "Channel out"=w3928:refnum<class "Channel.lvclass">)  [unwired: 7 in]
                n1765 = call-dynamic "Read State Machine.vi"("error in (no error)"=w3926, "Device in"=w3928) -> ("error out"=w3961:errorcluster, "State Machine.lvclass"=w3971:refnum<class "State Machine.lvclass">, "Device out"=w3970:refnum<class "Channel.lvclass">)  [unwired: 7 in]
                n1766 = call-dynamic "Write State.vi"("error in (no error)"=w3961, "State"=60, "State Machine in"=w3971) -> ("error out"=w3962:errorcluster, "State Machine out"=w3972:refnum<class "State Machine.lvclass">)  [unwired: 7 in]
                n1767 = call-dynamic "Write State Machine.vi"("error in (no error)"=w3962, "State Machine.lvclass"=w3972, "Device in"=w3970) -> ("error out"=w3974:errorcluster, "Device out"=w3973:refnum<class "Channel.lvclass">)  [unwired: 7 in]
                n1768 = call-dynamic "Write Channel.vi"("error in (no error)"=w3974, "Channel.lvclass"=w3973, "Acquisition in"=w3951) -> ("error out"=w3946:errorcluster, "Acquisition out"=w3947:refnum<class "Acquisition.lvclass">)  [unwired: 7 in]
              }
            }
            n1769 = case shown="True" w3812 {
              tunnel: w3814 -> [w3836 w3876]
              tunnel: w3813 -> [w3835 w3875]
              tunnel: [w3836 w3874] -> w3828
              tunnel: [w3835 w3873] -> w3827
              tunnel: w3805 -> [_ w3852]
              tunnel: w3804 -> [_ w3851]
              tunnel: w3803 -> [_ w3850]
              tunnel: w3802 -> [_ w3843]
              tunnel: w3801 -> [_ w3842]
              frame False {
              }
              frame True {
                # "nome do arquivo .cfg"
                # "seção no arquivo .cfg"
                n1770 = call-dynamic "Read Channel.vi"("error in (no error)"=w3875, "Acquisition in"=w3876) -> ("error out"=w3898:errorcluster, "Channel.lvclass"=w3899:refnum<class "Channel.lvclass">, "Acquisition out"=w3900:refnum<class "Acquisition.lvclass">)  [unwired: 7 in]
                n1771 = call-dynamic "Read Interface.vi"("error in (no error)"=w3898, "Channel in"=w3899) -> ("error out"=w3840:errorcluster, "Interface.lvclass"=w3838:refnum<class "Interface.lvclass">, "Channel out"=w3901:refnum<class "Channel.lvclass">)  [unwired: 7 in]
                n1772 = call-dynamic "Write restoreExpTime.vi"("error in (no error)"=w3840, "restoreExpTime"=TRUE, "Interface in"=w3838) -> ("error out"=w3839:errorcluster, "Interface out"=w3837:refnum<class "Interface.lvclass">)  [unwired: 7 in]
                n1773 = call-dynamic "Get CCD_Config.vi"("error in (no error)"=w3839, "Interface in"=w3837) -> ("error out"=w3846:errorcluster, "output cluster"=w3849:T24, "Interface out"=w3845:refnum<class "Interface.lvclass">)  [unwired: 7 in]
                n1774 = stacked-sequence {
                  tunnel: w3849 -> [_ w3907]
                  tunnel: [_ w3906] -> w3894
                  tunnel: w3849 -> [w3903 _]
                  tunnel: [w3902 _] -> w3844
                  frame #0 {
                    n1775 = Unbundle By Name(w3903) -> ("FRAME_TRANSFER"=w3902:bool)
                  }
                  frame #1 {
                    # "closed"
                    n1776 = Bundle By Name(cluster=w3907, "SHUTTER_MODE"=u8 2, "FRAME_TRANSFER"=FALSE) -> (w3906:T24)
                  }
                }
                n1777 = call-dynamic "Write PREV_FT.vi"("error in (no error)"=w3846, "PREV_FT"=w3844, "Interface in"=w3845) -> ("error out"=w3847:errorcluster, "Interface out"=w3848:refnum<class "Interface.lvclass">)  [unwired: 7 in]
                n1778 = call-dynamic "Set CCD_Config.vi"("error in (no error)"=w3847, "input cluster"=w3894, "Interface in"=w3848) -> ("error out"=w3895:errorcluster, "Interface out"=w3893:refnum<class "Interface.lvclass">)  [unwired: 7 in]
                n1779 = Flatten To String(anything=w3894, error in (no error)=w3895) -> (data string=w3897:string, error out=w3896:errorcluster)  [unwired: 2 in, 1 out]
                n1780 = call "Write flatted cluster.vi"("error in (no error)"=w3896, "flatted cluster"=w3897, "Interface in"=w3893) -> ("error out"=w3891:errorcluster, "Interface out"=w3892:refnum<class "Interface.lvclass">)  [unwired: 7 in]
                n1781 = call-dynamic "Write Interface.vi"("error in (no error)"=w3891, "Interface.lvclass"=w3892, "Channel in"=w3901) -> ("error out"=w3886:errorcluster, "Channel out"=w3885:refnum<class "Channel.lvclass">)  [unwired: 7 in]
                n1782 = call "Write section_name.vi"("error in (no error)"=w3886, "section_name"="CCD_ACS4", "Channel in"=w3885) -> ("error out"=w3887:errorcluster, "Channel out"=w3882:refnum<class "Channel.lvclass">)  [unwired: 7 in]
                n1783 = call-dynamic "save config.vi"("error in (no error)"=w3887, "file config"="lastsaved.cfg", "Channel in"=w3882) -> ("error out"=w3855:errorcluster, "Channel out"=w3856:refnum<class "Channel.lvclass">)  [unwired: 7 in]
                n1784 = local read "Filter4"() -> (w3872:u8)
                n1785 = call-dynamic "Write Filter.vi"("error in (no error)"=w3855, "Filter"=w3872, "Channel in"=w3856) -> ("error out"=w3865:errorcluster, "Channel out"=w3864:refnum<class "Channel.lvclass">)  [unwired: 7 in]
                n1786 = call-dynamic "Read Interface.vi"("error in (no error)"=w3865, "Channel in"=w3864) -> ("error out"=w3867:errorcluster, "Interface.lvclass"=w3862:refnum<class "Interface.lvclass">, "Channel out"=w3863:refnum<class "Channel.lvclass">)  [unwired: 7 in]
                n1787 = call-dynamic "Write Suffix.vi"("error in (no error)"=w3867, "Suffix"=w3843, "Interface in"=w3862) -> ("error out"=w3871:errorcluster, "Interface out"=w3861:refnum<class "Interface.lvclass">)  [unwired: 7 in]
                n1788 = call-dynamic "Write ObsType.vi"("error in (no error)"=w3871, "ObsType"=w3842, "Interface in"=w3861) -> ("error out"=w3870:errorcluster, "Interface out"=w3860:refnum<class "Interface.lvclass">)  [unwired: 7 in]
                n1789 = call-dynamic "Write Object.vi"("error in (no error)"=w3870, "Object"=w3850, "Interface in"=w3860) -> ("error out"=w3869:errorcluster, "Interface out"=w3859:refnum<class "Interface.lvclass">)  [unwired: 7 in]
                n1790 = call-dynamic "Write Comments.vi"("error in (no error)"=w3869, "Comments"=w3851, "Interface in"=w3859) -> ("error out"=w3868:errorcluster, "Interface out"=w3858:refnum<class "Interface.lvclass">)  [unwired: 7 in]
                n1791 = call-dynamic "Write Observer.vi"("error in (no error)"=w3868, "Observer"=w3852, "Interface in"=w3858) -> ("error out"=w3866:errorcluster, "Interface out"=w3857:refnum<class "Interface.lvclass">)  [unwired: 7 in]
                n1792 = call-dynamic "Write Interface.vi"("error in (no error)"=w3866, "Interface.lvclass"=w3857, "Channel in"=w3863) -> ("error out"=w3854:errorcluster, "Channel out"=w3853:refnum<class "Channel.lvclass">)  [unwired: 7 in]
                n1793 = call-dynamic "Read State Machine.vi"("error in (no error)"=w3854, "Device in"=w3853) -> ("error out"=w3890:errorcluster, "State Machine.lvclass"=w3880:refnum<class "State Machine.lvclass">, "Device out"=w3881:refnum<class "Channel.lvclass">)  [unwired: 7 in]
                n1794 = call-dynamic "Write State.vi"("error in (no error)"=w3890, "State"=60, "State Machine in"=w3880) -> ("error out"=w3889:errorcluster, "State Machine out"=w3879:refnum<class "State Machine.lvclass">)  [unwired: 7 in]
                n1795 = call-dynamic "Write State Machine.vi"("error in (no error)"=w3889, "State Machine.lvclass"=w3879, "Device in"=w3881) -> ("error out"=w3877:errorcluster, "Device out"=w3878:refnum<class "Channel.lvclass">)  [unwired: 7 in]
                n1796 = call-dynamic "Write Channel.vi"("error in (no error)"=w3877, "Channel.lvclass"=w3878, "Acquisition in"=w3900) -> ("error out"=w3873:errorcluster, "Acquisition out"=w3874:refnum<class "Acquisition.lvclass">)  [unwired: 7 in]
              }
            }
            n1797 = property on="Exptime ch1" class="DigNum (strict)"("Value"=w3824) -> ()  [unwired: 2 in, 2 out]
            n1798 = property on="Exptime ch2" class="DigNum (strict)"("Value"=w3824) -> ()  [unwired: 2 in, 2 out]
            n1799 = property on="Exptime ch3" class="DigNum (strict)"("Value"=w3824) -> ()  [unwired: 2 in, 2 out]
            n1800 = property on="Exptime ch4" class="DigNum (strict)"("Value"=w3824) -> ()  [unwired: 2 in, 2 out]
          }
          frame "DARK" {
            # "DARK: Shutter automatically closed and restore FRAME_TRANSFER."
            n1801 = call "Read connection.vi"("error in (no error)"=w4132, "Server in"=w4133) -> ("error out"=w4139:errorcluster, "connection"=w4138:bool, "Server out"=w4140:refnum<class "Acquisition.lvclass">)  [unwired: 7 in]
            n1802 = call "Read connection.vi"("error in (no error)"=w4136, "Server in"=w4137) -> ("error out"=w4145:errorcluster, "connection"=w4144:bool, "Server out"=w4146:refnum<class "Acquisition.lvclass">)  [unwired: 7 in]
            n1803 = call "Read connection.vi"("error in (no error)"=w4134, "Server in"=w4135) -> ("error out"=w4142:errorcluster, "connection"=w4141:bool, "Server out"=w4143:refnum<class "Acquisition.lvclass">)  [unwired: 7 in]
            n1804 = call "Read connection.vi"("error in (no error)"=w4150, "Server in"=w4151) -> ("error out"=w4148:errorcluster, "connection"=w4147:bool, "Server out"=w4149:refnum<class "Acquisition.lvclass">)  [unwired: 7 in]
            n1805 = case shown="True" w4138 {
              tunnel: w4140 -> [w4161 w4201]
              tunnel: w4139 -> [w4160 w4200]
              tunnel: [w4161 w4199] -> w4153
              tunnel: [w4160 w4198] -> w4152
              tunnel: w4131 -> [_ w4176]
              tunnel: w4130 -> [_ w4175]
              tunnel: w4129 -> [_ w4174]
              tunnel: w4128 -> [_ w4168]
              tunnel: w4127 -> [_ w4167]
              frame False {
              }
              frame True {
                # "nome do arquivo .cfg"
                # "seção no arquivo .cfg"
                # "closed"
                n1806 = call-dynamic "Read Channel.vi"("error in (no error)"=w4200, "Acquisition in"=w4201) -> ("error out"=w4226:errorcluster, "Channel.lvclass"=w4227:refnum<class "Channel.lvclass">, "Acquisition out"=w4228:refnum<class "Acquisition.lvclass">)  [unwired: 7 in]
                n1807 = call-dynamic "Read Interface.vi"("error in (no error)"=w4226, "Channel in"=w4227) -> ("error out"=w4166:errorcluster, "Interface.lvclass"=w4165:refnum<class "Interface.lvclass">, "Channel out"=w4229:refnum<class "Channel.lvclass">)  [unwired: 7 in]
                n1808 = call-dynamic "Read restoreExpTime.vi"("error in (no error)"=w4166, "Interface in"=w4165) -> ("error out"=w4163:errorcluster, "restoreExpTime"=w4162:bool, "Interface out"=w4164:refnum<class "Interface.lvclass">)  [unwired: 7 in]
                n1809 = case shown="True" w4162 {
                  tunnel: w4164 -> [w4231 w4236]
                  tunnel: w4163 -> [w4230 w4234]
                  tunnel: [w4230 w4239] -> w4170
                  tunnel: [w4231 w4238] -> w4169
                  frame False {
                  }
                  frame True {
                    n1810 = call-dynamic "Write restoreExpTime.vi"("error in (no error)"=w4234, "restoreExpTime"=FALSE, "Interface in"=w4236) -> ("error out"=w4232:errorcluster, "Interface out"=w4235:refnum<class "Interface.lvclass">)  [unwired: 7 in]
                    n1811 = call-dynamic "Read prev ExpTime.vi"("error in (no error)"=w4232, "Interface in"=w4235) -> ("error out"=w4239:errorcluster, "prev ExpTime"=w4237:dbl, "Interface out"=w4238:refnum<class "Interface.lvclass">)  [unwired: 7 in]
                    n1812 = property on="Exptime ch4" class="DigNum (strict)"("Value"=w4237) -> ()  [unwired: 2 in, 2 out]
                  }
                }
                n1813 = call-dynamic "Read PREV_FT.vi"("error in (no error)"=w4170, "Interface in"=w4169) -> ("error out"=w4172:errorcluster, "PREV_FT"=w4171:bool, "Interface out"=w4173:refnum<class "Interface.lvclass">)  [unwired: 7 in]
